vi "Generate_Model_Name_and_Info(CSV).vi"(7 "Iteration_idx":i32, 10 "DS_Name":string, 11 "Model_Info_and_Report":T1 {"Eval Stats(Pixel)"."Recall(F1_Max)" format="%#.5f"; "Eval Stats(Pixel)"."FPR(F1_Max)" format="%#.5f"; "Eval Stats(Pixel)"."FNR(F1_Max)" format="%#.5f"; "Eval Stats(Pixel)"."Prec.(F1_Max)" format="%#.5f"; "Eval Stats(Pixel)"."F1_Max" format="%#.5f"; "Eval Stats(Pixel)"."AUROC" format="%#.5f"; "Eval Stats(Pixel)"."Scores(Bad)"."Min" format="%#_5g"; "Eval Stats(Pixel)"."Scores(Good)"."Min" format="%#_5g"; "Eval Stats(Pixel)"."Thrshld(F1_Max)" format="%#_5f"; "Eval Stats(Image)"."Recall(F1_Max)" format="%#.5f"; "Eval Stats(Image)"."FPR(F1_Max)" format="%#.5f"; "Eval Stats(Image)"."FNR(F1_Max)" format="%#.5f"; "Eval Stats(Image)"."Prec.(F1_Max)" format="%#.5f"; "Eval Stats(Image)"."F1_Max" format="%#.5f"; "Eval Stats(Image)"."AUROC" format="%#.5f"; "Eval Stats(Image)"."Scores(Bad)"."Min" format="%#_5g"; "Eval Stats(Image)"."Scores(Good)"."Min" format="%#_5g"; "Eval Stats(Image)"."Thrshld(F1_Max)" format="%#_5f"}) -> (2 "Model_Info(CSV)":string, 3 "Generated_Model_Name":string)   [LabVIEW 2020]
uses:
  Controls/Model_Info_and_Report.ctl
  <vilib>/Ngene/Deep Learning Toolkit/Toolkit/NN_Data/API/NN_Dims(C,H,W).ctl
  Controls/Feature_Layers_CFG.ctl
  <vilib>/Ngene/DeepLTK Anomaly Detection Addon/Toolkit/API/Controls/Eval_Results.ctl
  <vilib>/Ngene/DeepLTK Anomaly Detection Addon/Toolkit/API/Controls/MinMax.ctl
  <vilib>/Ngene/DeepLTK Anomaly Detection Addon/Toolkit/DeepLTK_Anomaly_Detection_Addon.lvlib
  <vilib>/Ngene/Deep Learning Toolkit/Toolkit/Deep_Learning_Toolkit_by_Ngene.lvlib
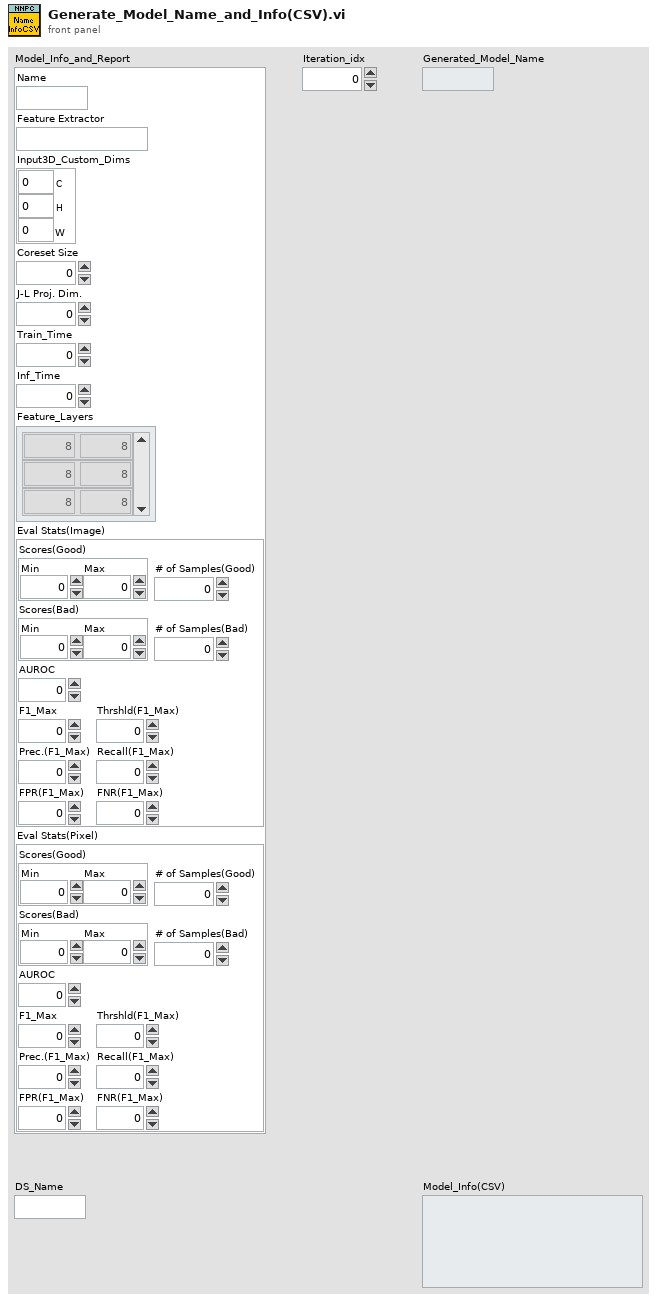
[diagram p1: front panel]
types:
  T1 = typedef "Model_Info_and_Report.ctl" = cluster{"Name":string, "Feature Extractor":string, "Input3D_Custom_Dims":T2, "Coreset Size":i32, "J-L Proj. Dim.":i32, "Train_Time":dbl, "Inf_Time":dbl, "Feature_Layers":T3, "Eval Stats(Image)":T4, "Eval Stats(Pixel)":T4}
  T2 = typedef "Deep_Learning_Toolkit_by_Ngene.lvlib/NN_Dims(C,H,W).ctl" = cluster{"C":i32, "H":i32, "W":i32}
  T3 = typedef "Feature_Layers_CFG.ctl" = cluster{"Layer_ID":i32, "Patch_Size":i32}[]
  T4 = typedef "DeepLTK_Anomaly_Detection_Addon.lvlib/Eval_Results.ctl" = cluster{"Scores(Good)":T5, "Scores(Bad)":T5, "# of Samples(Good)":i32, "# of Samples(Bad)":i32, "AUROC":sgl, "F1_Max":sgl, "Thrshld(F1_Max)":sgl, "Prec.(F1_Max)":sgl, "Recall(F1_Max)":sgl, "FPR(F1_Max)":sgl, "FNR(F1_Max)":sgl}
  T5 = typedef "DeepLTK_Anomaly_Detection_Addon.lvlib/MinMax.ctl" = cluster{"Min":sgl, "Max":sgl}
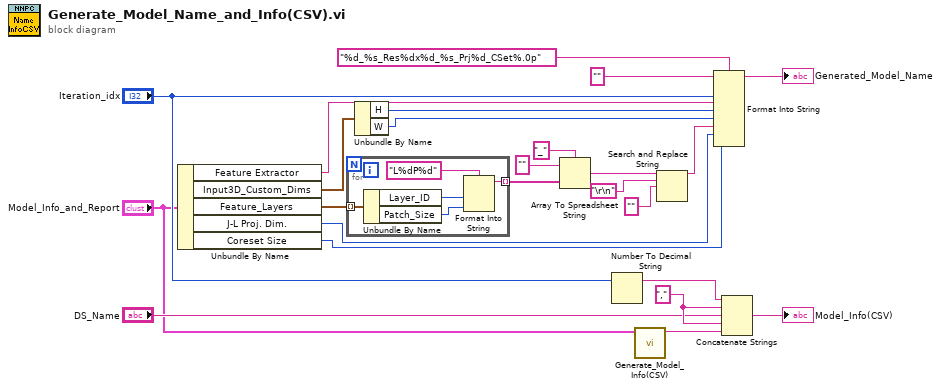
[diagram p0: block diagram]
diagram:
  w6 = "," ("string")
  n1 = Unbundle By Name("Model_Info_and_Report") -> ("Feature Extractor"=w18:string, "Input3D_Custom_Dims"=w10:T2, "Feature_Layers"=w12:T3, "J-L Proj. Dim."=w16:i32, "Coreset Size"=w17:i32)
  n2 = for {
    tunnel: w12 -> [w29] mode=indexing
    tunnel: [w25] -> w15 mode=indexing
    n3 = Unbundle By Name(w29) -> ("Layer_ID"=w28:i32, "Patch_Size"=w27:i32)
    n4 = Format Into String(format string="L%dP%d", w28, w27) -> (resulting string=w25:string)  [unwired: 2 in, 1 out]
  }
  n5 = Unbundle By Name(w10) -> ("H"=w11:i32, "W"=w24:i32)
  n6 = Array To Spreadsheet String(delimiter (Tab)="_", array=w15, 3:"" ("format string")) -> (spreadsheet string=w22:string)
  n7 = Number To Decimal String(number="Iteration_idx") -> (decimal integer string=w4:string)  [unwired: 1 in]
  n8 = call "Generate_Model_Info(CSV).vi"("Model_Info_and_Report"="Model_Info_and_Report") -> ("Model_Info(CSV)"=w7:string)  [unwired: 10 in]
  n9 = Search and Replace String(input string=w22, search string="\r\n", replace string="" ("replace string (\"\")")) -> (result string=w23:string)  [unwired: 5 in, 3 out]
  n10 = Format Into String(format string="%d_%s_Res%dx%d_%s_Prj%d_CSet%.0p", initial string="", "Iteration_idx", w18, w11, w24, w23, w16, w17) -> (resulting string=→"Generated_Model_Name":string)  [unwired: 1 in, 1 out]
  n11 = Concatenate Strings(w4, w6, "DS_Name", w6, w7) -> (→"Model_Info(CSV)":string)
